vi "create_collection.vi"(0 "vector_qdrant in":refnum<class "vector_qdrant.lvclass">, 5 "collection_name":string, 7 "vector_size":u32, 9 "distance":string, 11 "error in (no error)":errorcluster) -> (4 "vector_qdrant out":refnum<class "vector_qdrant.lvclass">, 15 "error out":errorcluster)   [LabVIEW 2020, in "vector_qdrant.lvclass"]
uses:
  vector_qdrant.lvclass
  vector_qdrant.lvclass/vector_qdrant.ctl
  <vilib>/httpClient/PUTBuffer.vi
  <vilib>/httpClient/LabVIEWHTTPClient.lvlib
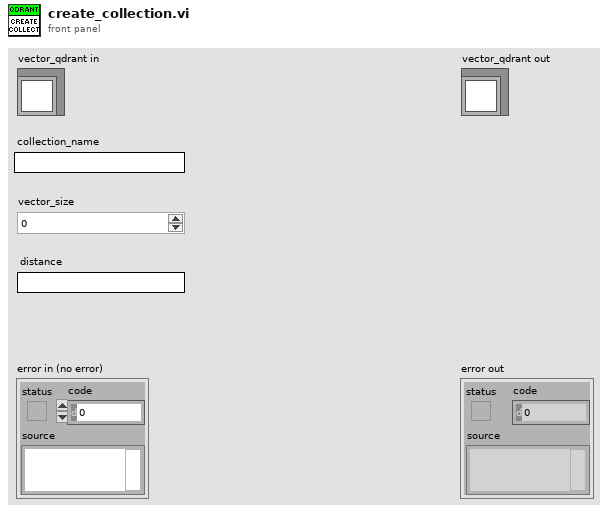
[diagram p1: front panel]
types:
  T1 = cluster{"vectors":cluster{"size":u32, "distance":string}}
  T2 = typedef "LabVIEWHTTPClient.lvlib/ClientHandle.ctl" = refnum<k1>
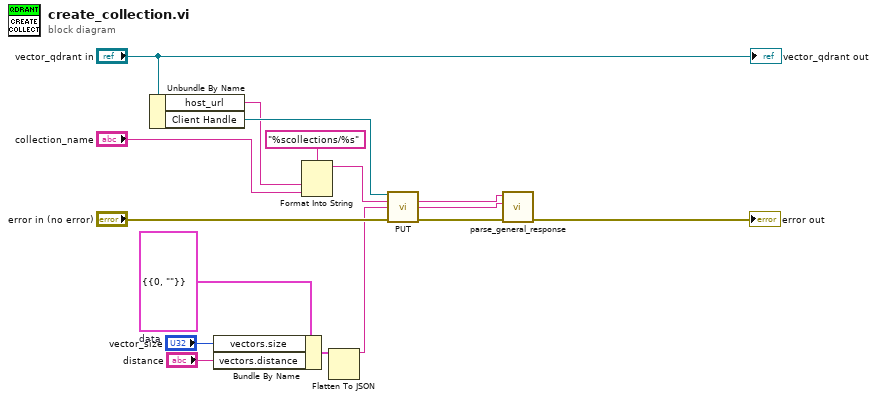
[diagram p0: block diagram]
diagram:
  w1 = T1 {"vectors"={"size"=0, "distance"=""}}  # data
  n1 = Unbundle By Name("vector_qdrant in") -> ("host_url"=w13:string, "Client Handle"=w15:T2)
  n2 = Bundle By Name(cluster=w1, "vectors.size"="vector_size", "vectors.distance"="distance") -> (w8:T1)
  n3 = Format Into String(format string="%scollections/%s", w13, "collection_name") -> (resulting string=w11:string)  [unwired: 2 in, 1 out]
  n4 = Flatten To JSON(anything=w8) -> (JSON string=w7:string)  [unwired: 2 in, 1 out]
  n5 = call-poly <vilib>:"PUT.vi"("client handle"=w15, "url"=w11, "buffer"=w7, "error in (no error)"="error in (no error)") -> ("headers"=w3:string, "body"=w2:string, "error out"=w5:errorcluster)  [unwired: 8 in, 1 out]
  n6 = call "parse_general_response.vi"("error in (no error)"=w5, "body"=w2, "headers"=w3) -> ("error out"=→"error out":errorcluster)  [unwired: 8 in]
  "vector_qdrant out" <- "vector_qdrant in"
